vi "getSerializedData.vi"(0 "reference":refnum<class "ActorNode.lvclass">, 5 "error in (no error)":errorcluster) -> (14 "reference out":refnum<class "ActorNode.lvclass">, 15 "parent":refnum<class "AbstractNode.lvclass">, 16 "children":refnum<class "AbstractNode.lvclass">[](array[class]), 17 "xmlOut":string, 19 "error out":errorcluster)   [LabVIEW 2012, in "ActorNode.lvclass"]
doc: "getSerializedData"
uses:
  <resource>/Framework/Providers/Open_GDS/UML/ActorNode_class/ActorNode.lvclass
  <resource>/Framework/Providers/Open_GDS/UML/AbstractNode_class/AbstractNode.lvclass
  <resource>/Framework/Providers/Open_GDS/UML/AbstractNode_class/ObjectReference.ctl
  <resource>/Framework/Providers/Open_GDS/UML/General/Rectangle/Rectangle Rectangle2D.ctl
  <resource>/Framework/Providers/Open_GDS/UML/MultiLineString_class/ObjectReference.ctl
  <resource>/Framework/Providers/Open_GDS/UML/MultiLineString_class/MultiLineString.lvclass
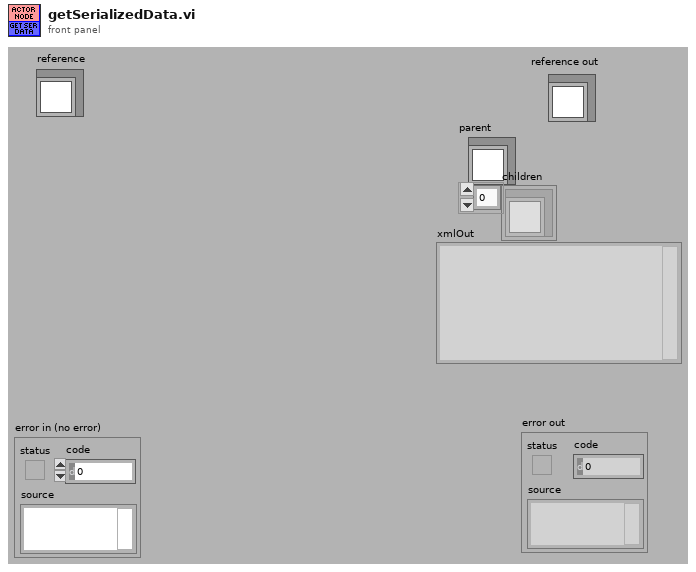
[diagram p1: front panel]
types:
  T1 = typedef "AbstractNode.lvclass/ObjectReference.ctl" = refnum<k1>
  T2 = typedef "Rectangle Rectangle2D.ctl" = cluster{"x":dbl, "y":dbl, "width":dbl, "height":dbl}
  T3 = typedef "MultiLineString.lvclass/ObjectReference.ctl" = refnum<k1>
  T4 = cluster{"Base class":cluster{"Base class":cluster{"parent":T1, "children":T1[]}, "bounds":T2}, "name":T3, "DEFAULT_WIDTH":i32, "DEFAULT_HEIGHT":i32, "DEFAULT_GAP":i32}
  T5 = typedef "ActorNode.lvclass/ObjectAttributes.ctl" = cluster{"Base class":T6, "name":refnum<class "MultiLineString.lvclass">, "DEFAULT_WIDTH":i32, "DEFAULT_HEIGHT":i32, "DEFAULT_GAP":i32}
  T6 = typedef "RectangularNode.lvclass/ObjectAttributes.ctl" = cluster{"Base class":T7, "bounds":T2}
  T7 = typedef "AbstractNode.lvclass/ObjectAttributes.ctl" = cluster{"parent":refnum<class "AbstractNode.lvclass">, "children":refnum<class "AbstractNode.lvclass">[], "Hidden":bool}
  T8 = cluster{"Attributes":cluster{"Base class":cluster{"Base class":cluster{"parent":T1, "children":T1[]}, "bounds":T2}, "name":T3, "DEFAULT_WIDTH":i32, "DEFAULT_HEIGHT":i32, "DEFAULT_GAP":i32}, "text":string}
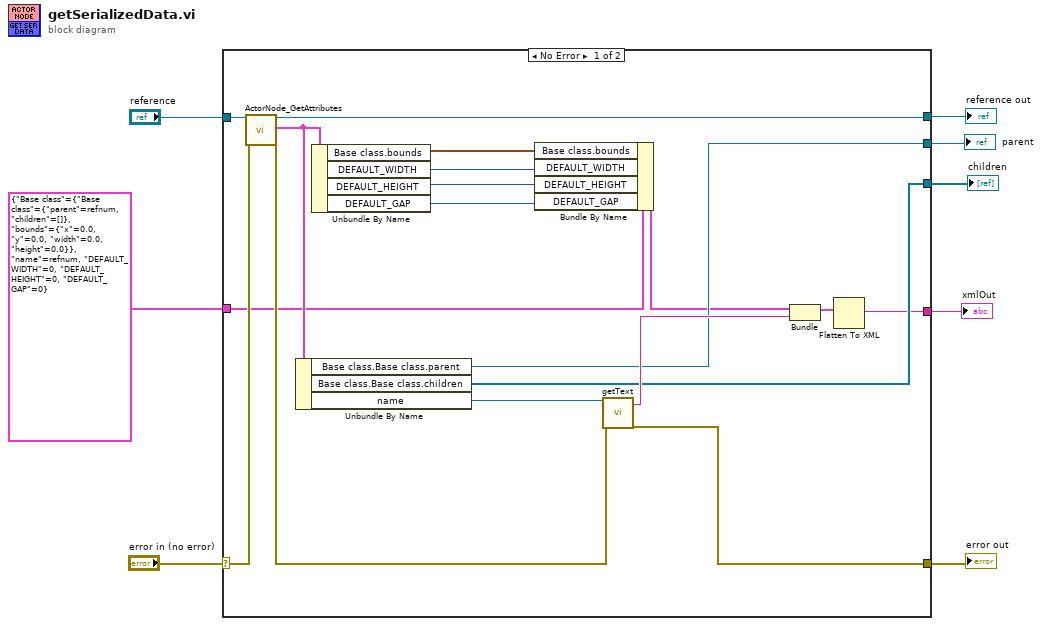
[diagram p0: block diagram]
diagram:
  n1 = case shown="No Error" "error in (no error)" {
    selector: "error in (no error)" -> [w26 w27]
    tunnel: "reference" -> [w25 w28]
    tunnel: [w16 w27] -> w6
    tunnel: [w24 w28] -> w5
    tunnel: [w19 _] -> w4
    tunnel: [w18 _] -> w3
    tunnel: [w17 _] -> w2
    tunnel: T4 {"Base class"={"Base class"={"parent"=refnum, "children"=[]}, "bounds"={"x"=0.0, "y"=0.0, "width"=0.0, "height"=0.0}}, "name"=refnum, "DEFAULT_WIDTH"=0, "DEFAULT_HEIGHT"=0, "DEFAULT_GAP"=0} ("Attributes") -> [w14 _]
    frame No Error {
      n2 = call <resource>:"ActorNode_GetAttributes.vi"("reference in"=w25, "error in (no error)"=w26) -> ("reference out"=w24:refnum<class "ActorNode.lvclass">, "Attributes"=w15:T5, "error out"=w20:errorcluster)  [unwired: 15 out]
      n3 = Unbundle By Name(w15) -> ("Base class.Base class.parent"=w19:refnum<class "AbstractNode.lvclass">, "Base class.Base class.children"=w18:refnum<class "AbstractNode.lvclass">[], "name"=w22:refnum<class "MultiLineString.lvclass">)
      n4 = Unbundle By Name(w15) -> ("Base class.bounds"=w12:T2, "DEFAULT_WIDTH"=w11:i32, "DEFAULT_HEIGHT"=w10:i32, "DEFAULT_GAP"=w9:i32)
      n5 = Bundle By Name(cluster=w14, "Base class.bounds"=w12, "DEFAULT_WIDTH"=w11, "DEFAULT_HEIGHT"=w10, "DEFAULT_GAP"=w9) -> (w13:T4)
      n6 = call-dynamic "getText.vi"("reference"=w22, "error in (no error)"=w20) -> ("text"=w21:string, "error out"=w16:errorcluster)  [unwired: 16 out]
      n7 = Bundle("Attributes"=w13, "text"=w21) -> (w23:T8)  [unwired: 1 out]
      n8 = Flatten To XML(anything=w23) -> (xml string=w17:string)
    }
    frame Error {
    }
  }
  "reference out" <- w5
  "error out" <- w6
  "parent" <- w4
  "children" <- w3
  "xmlOut" <- w2
